vi "Go To Work.vi"(8 "error in (no error)":errorcluster, 11 "Work in":refnum<class "Work.lvclass">) -> (0 "error out":errorcluster, 3 "State Actor.lvclass":refnum<class "State Actor.lvclass">)   [LabVIEW 2024, in "Test States.lvlib" / "Work.lvclass"]
uses:
  Work.lvclass
  Work.lvclass/Work.ctl
  <vilib>/ni/Actors/State Actor/State Actor/State Actor.lvclass
  G:/Leveling/LabVIEW/Learning/Actor Framework/actor-state-machine/Test States/Test State/Test State.lvclass
  C:/Program Files/National Instruments/LabVIEW 2024/vi.lib/ni/Actors/State Actor/State Actor/State Actor.lvclass
  C:/Program Files/National Instruments/LabVIEW 2024/vi.lib/ActorFramework/Actor/Actor.lvclass
  G:/Leveling/LabVIEW/Learning/Actor Framework/actor-state-machine/Test States/Work/Work.lvclass
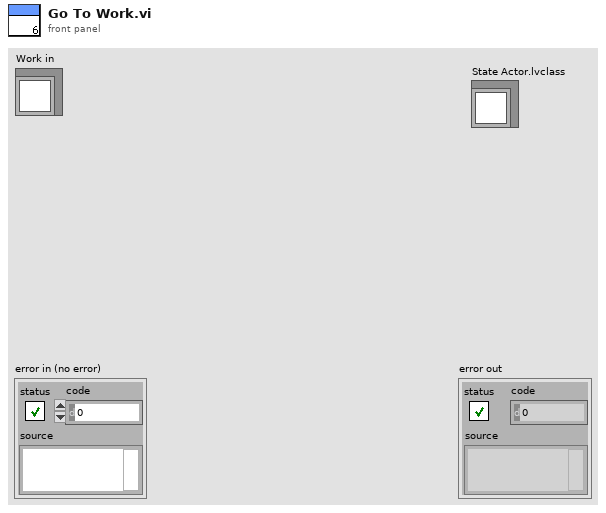
[diagram p1: front panel]
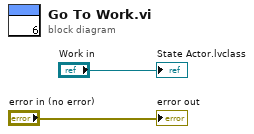
[diagram p0: block diagram]
diagram:
  "error out" <- "error in (no error)"
  "State Actor.lvclass" <- "Work in"
